vi "Init_Test.vi"(8 "error in (no error)":errorcluster caption="entrée d'erreur (pas d'erreur)", 11 "Nodon_Check_ZCR_Calibration en entrée":refnum<class "Nodon_Check_ZCR_Calibration.lvclass">) -> (0 "error out":errorcluster caption="sortie d'erreur", 3 "Nodon_Check_ZCR_Calibration en sortie":refnum<class "Nodon_Check_ZCR_Calibration.lvclass">)   [LabVIEW 2020, in "Library Test.lvlib" / "Nodon_Check_ZCR_Calibration.lvclass"]
uses:
  Nodon_Check_ZCR_Calibration.lvclass
  C:/Users/ngarcin/OneDrive - Altyor/Standard TB/Class/Test/Test (Default)/Test (Default).lvclass
  Commun VI/TypeDef/Commande Test/Commande Type Test.ctl
  Commun VI/TypeDef/Commande Test/Commande Value Type.ctl
  Test_Without_Instr/Test_Without_Inst.lvclass
  Nodon_Check_ZCR_Calibration.lvclass/Nodon_Check_ZCR_Calibration.ctl
  Commun VI/Library Commun.lvlib
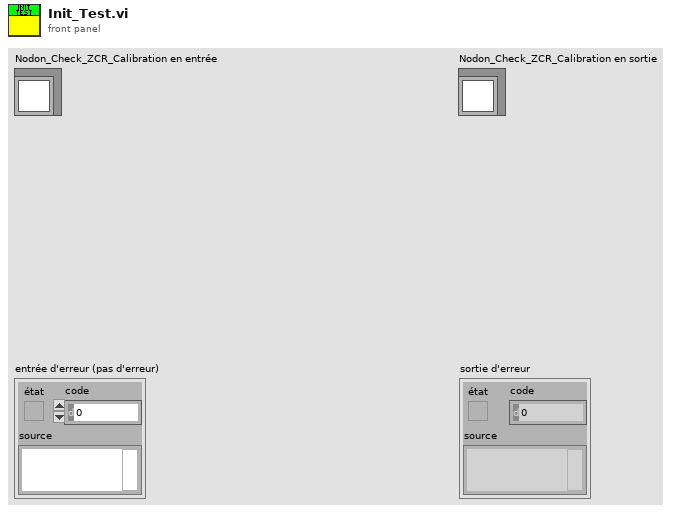
[diagram p1: front panel]
types:
  T1 = typedef "Library Commun.lvlib/Commande Value Type.ctl" = enum16{"None", "String", "Number", "Timestamp", "Boolean", "Array"}
  T2 = typedef "Library Commun.lvlib/Commande Type Test.ctl" = enum16{"Function", "Test", "Calculation"}
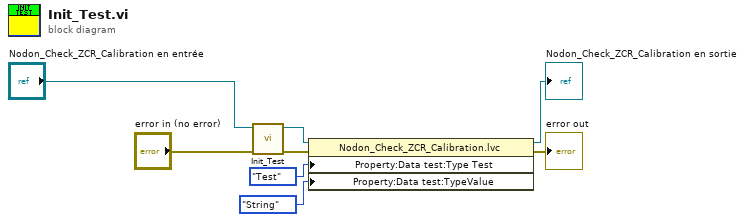
[diagram p0: block diagram]
diagram:
  n1 = call-parent "Init_Test.vi"("error in (no error)"="error in (no error)", "Test_Without_Inst en entrée"="Nodon_Check_ZCR_Calibration en entrée") -> ("error out"=w6:errorcluster, "Test_Without_Inst en sortie"=w7:refnum<class "Nodon_Check_ZCR_Calibration.lvclass">)  [unwired: 8 in]
  n2 = property class="Nodon_Check_ZCR_Calibration.lvc"(reference=w7, error in=w6, "Property:Data test:Type Test"=Commande_Type_Test."Test" ("Type Test"), "Property:Data test:TypeValue"=Commande_Value_Type."String" ("TypeValue")) -> (reference out=→"Nodon_Check_ZCR_Calibration en sortie":refnum<class "Nodon_Check_ZCR_Calibration.lvclass">, error out=→"error out":errorcluster)
